vi "DAQ Multi IO Init.vi"(8 "error in":errorcluster) -> (0 "error out":errorcluster, 3 "DAQ Ref Cluster":T1)   [LabVIEW 2021]
uses:
  Muscle Actuator/Muscle Actuator LabV Analog/Controls/DAQ Refnums.ctl
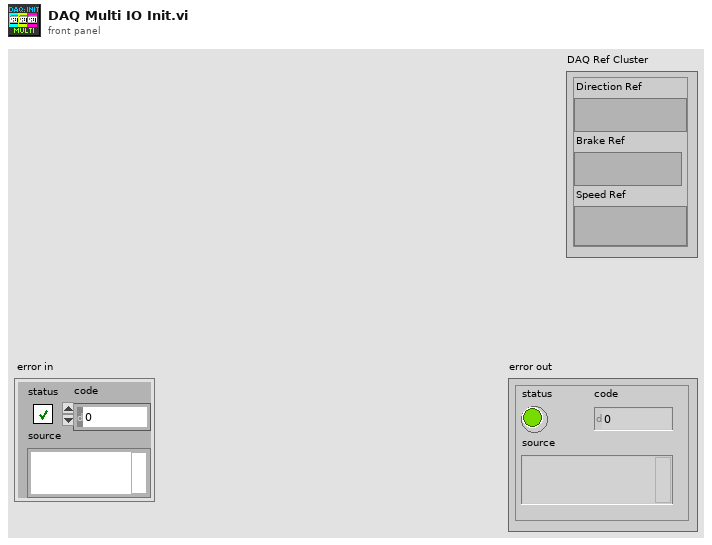
[diagram p1: front panel]
types:
  T1 = typedef "DAQ Refnums.ctl" = cluster{"Direction Ref":refnum<k21>, "Brake Ref":refnum<k21>, "Speed Ref":refnum<k21>}
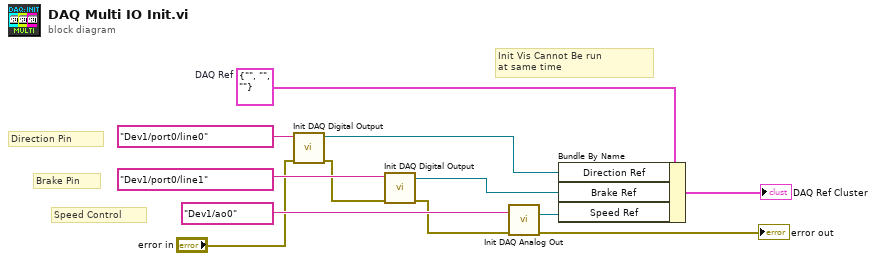
[diagram p0: block diagram]
diagram:
  w12 = T1 {"Direction Ref"="", "Brake Ref"="", "Speed Ref"=""}  # DAQ Ref
  # "Init Vis Cannot Be run\nat same time"
  # "Speed Control"
  # "Direction Pin"
  # "Brake Pin"
  n1 = call "Init DAQ Digital Output.vi"("error in"="error in", "lines"=tag "Dev1/port0/line0") -> ("error out"=w5:errorcluster, "Refnum out"=w8:refnum<k21>)  [unwired: 8 in]
  n2 = call "Init DAQ Digital Output.vi"("error in"=w5, "lines"=tag "Dev1/port0/line1") -> ("error out"=w2:errorcluster, "Refnum out"=w10:refnum<k21>)  [unwired: 8 in]
  n3 = call "Init DAQ Analog Out.vi"("error in"=w2, "physical channels"=tag "Dev1/ao0") -> ("error out"=→"error out":errorcluster, "Refnum out"=w9:refnum<k21>)  [unwired: 8 in]
  n4 = Bundle By Name(cluster=w12, "Direction Ref"=w8, "Brake Ref"=w10, "Speed Ref"=w9) -> (→"DAQ Ref Cluster":T1)
